vi "HWR.vi"() -> ()   [LabVIEW 2021]
panel:
  in  "stop":bool
  in  "Amp":dbl
  in  "Numeric":dbl
  out "Waveform Graph":dynamicdata(graph)
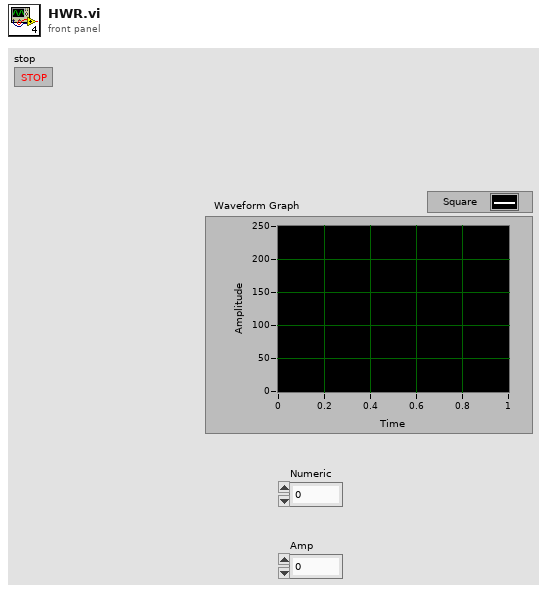
[diagram p1: front panel]
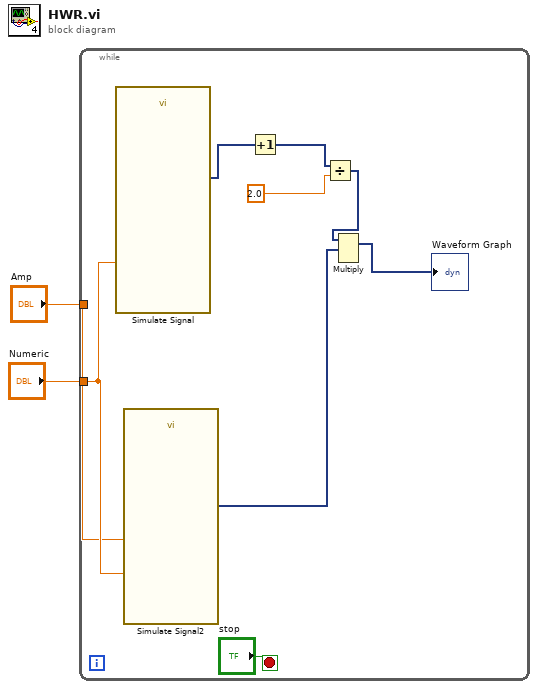
[diagram p0: block diagram]
diagram:
  n1 = while {
    tunnel: "Numeric" -> [w10]
    tunnel: "Amp" -> [w9]
    stop <- "stop" stop-if-true
    n2 = call "Simulate Signal"("Frequency"=w10) -> ("Square"=w11:dynamicdata)  [unwired: 13 in, 1 out]
    n3 = call "Simulate Signal2"("Frequency"=w10, "Amplitude"=w9) -> ("Sine"=w5:dynamicdata)  [unwired: 12 in, 1 out]
    n4 = Increment(x=w11) -> (x+1=w6:dynamicdata)
    n5 = Divide(x=w6, y=2.0) -> (x/y=w4:dynamicdata)
    n6 = Multiply(1:w5, 2:w4) -> (0:→"Waveform Graph":dynamicdata)  [unwired: 1 in, 1 out]
  }
